vi "PH_PILS.set Doors HV room.vi"(0 "i ref in":refnum<vi>, 2 "Service Name":string="N/A", 5 "error in":errorcluster) -> (14 "i ref out":refnum<vi>, 19 "error out":errorcluster)   [LabVIEW 2014, in "PH_PILS.lvlib"]
doc: "This VI sets the GUI elements related to the doors of the HV room."
uses:
  PH_PILS.lvlib
  PH_PILS.Operation Mode.ctl
  PH_PILS.Submode.ctl
  PH_Basics/PH_Common/PH_Common.lvlib
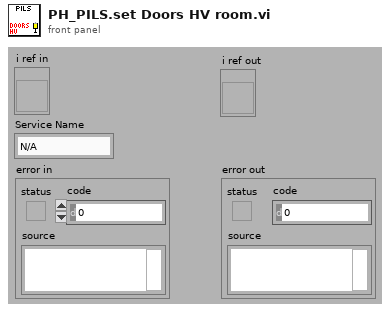
[diagram p1: front panel]
types:
  T1 = typedef "PH_PILS.lvlib/PH_PILS.Submode.ctl" = enum16{"unknown", "HV-Normal", "HV-Test"}
  T2 = typedef "PH_PILS.lvlib/PH_PILS.Operation Mode.ctl" = enum16{"unknown", "Service", "Labor", "Search", "Shot"}
  T3 = typedef "PH_PILS.lvlib/PH_PILS.i attribute.ctl" = cluster{"Boolean":cluster{"GUI Ref":refnum<vi>, "Status":i32}[], "GUI Refs Exp. Shutters":cluster{"1":refnum<vi>, "2":refnum<vi>, "3":refnum<vi>, "4":refnum<vi>}, "Tristate2Run GUI Refs":refnum<vi>[], "EO-Likes":cluster{"GUI Ref":refnum<vi>, "Status":i32}[], "Operation Mode":cluster{"Operation Mode":T2, "GUI":cluster{"Ref State":refnum<vi>, "Ref":refnum<vi>}, "Servicemode":cluster{"Tagname":string, "Status":i32}, "Labormode":cluster{"Tagname":string, "Status":i32}, "Searchmode":cluster{"Tagname":string, "Status":i32}, "Shotmode":cluster{"Tagname":string, "Status":i32}}, "Submode":cluster{"Submode":T1, "GUI":cluster{"Ref State":refnum<vi>, "Ref":refnum<vi>}, "Submode":cluster{"Tagname":string, "Status":i32}}, "Experiment":cluster{"Experiment":enum16{"unknown", "intern", "4 (Z6)", "3", "2", "1"}, "GUI":cluster{"Ref State":refnum<vi>, "Ref":refnum<vi>}, "intern":cluster{"Tagname":string, "Status":i32}, "Exp 4":cluster{"Tagname":string, "Status":i32}, "Exp 3":cluster{"Tagname":string, "Status":i32}, "Exp 2":cluster{"Tagname":string, "Status":i32}, "Exp 1":cluster{"Tagname":string, "Status":i32}}, "TristateNormal":cluster{"GUI Ref":refnum<vi>, "Status":i32}[], "Door Tags":cluster{"GUI Ref":refnum<vi>, "Status":i32}[], "GUIlessTags":cluster{"Name":string, "Status":i32}[], "Beamline GUI Refs":refnum<vi>[], "Special Boolean":cluster{"GUI Ref":refnum<vi>, "Status":i32}[], "Laserpower":cluster{"GUI Ref":refnum<vi>, "Status":i32}[], "Shutter":cluster{"GUI Ref":refnum<vi>, "Status":i32}[], "Tristate EO Like":cluster{"GUI Ref":refnum<vi>, "Status":i32}[], "PP":cluster{"GUI Ref":refnum<vi>, "Status":i32, "Head Ref":refnum<vi>, "Slider Ref":refnum<vi>}[], "Switch Knobs":cluster{"GUI Ref":refnum<vi>, "Status":i32}[], "Latch Knob GUI Refs":refnum<vi>[], "FailureCounter":i32, "Enabled Status":cluster{"Laser":i32, "PreAmp":i32, "MainAmp":i32}, "Mercury":refnum<vi>, "Instance Rods":string, "Logfile":path, "Beckhoff-Instance Internal":string, "Beckhoff-Instance External":string, "Enabling Rights":cluster{"Name":string, "Password":string, "PA?":bool, "MA?":bool, "Exp?":bool}[]}
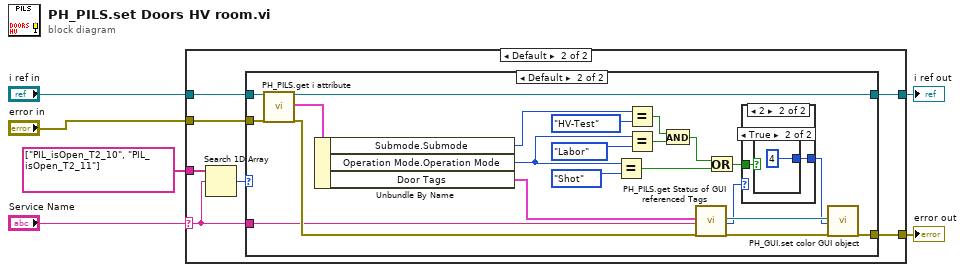
[diagram p0: block diagram]
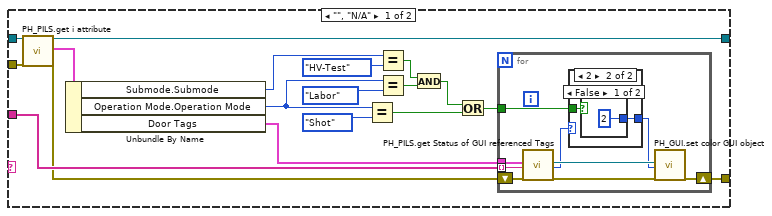
[diagram p2: hidden frame]
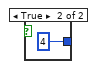
[diagram p4: hidden frame]
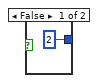
[diagram p7: hidden frame]
diagram:
  n1 = case shown="Default" "Service Name" {
    selector: "Service Name" -> [_ w40]
    tunnel: "error in" -> [w24 w45]
    tunnel: [w23 w44] -> w5
    tunnel: "i ref in" -> [w22 w43]
    tunnel: [w20 w42] -> w3
    tunnel: string[] ["PIL_isOpen_T2_10", "PIL_isOpen_T2_11"] -> [w19 w41]
    frame "", "N/A" {
      n2 = call "PH_PILS.get i attribute.vi"("i ref in"=w22, "error in (no error)"=w24) -> ("i ref out"=w23:refnum<vi>, "i attribute"=w21:T3, "error out"=w16:errorcluster)  [unwired: 15 in]
      n3 = Unbundle By Name(w21) -> ("Submode.Submode"=w13:T1, "Operation Mode.Operation Mode"=w14:T2, "Door Tags"=w17:cluster{"GUI Ref":refnum<vi>, "Status":i32}[])
      n4 = Equal?(x=w14, y=PH_PILS.Operation_Mode."Shot" ("Operation Mode.Operation Mode")) -> (x = y?=w8:bool)
      n5 = Equal?(x=w13, y=PH_PILS.Submode."HV-Test" ("Submode.Submode")) -> (x = y?=w11:bool)
      n6 = Equal?(x=w14, y=PH_PILS.Operation_Mode."Labor" ("Operation Mode.Operation Mode")) -> (x = y?=w10:bool)
      n7 = And(x=w11, y=w10) -> (x .and. y?=w9:bool)
      n8 = Or(x=w9, y=w8) -> (x .or. y?=w7:bool)
      n9 = for {
        tunnel: w17 -> [w33]
        tunnel: w19 -> [w30] mode=indexing
        shift-right: [w29] -> w20
        shift-left: w16 -> [w32]
        tunnel: w7 -> [w25]
        n10 = call "PH_PILS.get Status of GUI referenced Tags.vi"("Tags"=w33, "Tagname"=w30, "error in"=w32) -> ("GUI Ref"=w28:refnum<vi>, "Status"=w27:i32, "error out"=w31:errorcluster)  [unwired: 13 in, 1 out]
        n11 = case shown="2" w27 {
          selector: w27 -> [w34 _]
          tunnel: [w34 w36] -> w26
          tunnel: w25 -> [_ w35]
          frame 0, Default {
          }
          frame 2 {
            n12 = case shown="False" w35 {
              tunnel: [2 4] -> w36
              frame False {
              }
              frame True {
              }
            }
          }
        }
        n13 = call "PH_GUI.set color GUI object.vi"("GUI object Ref"=w28, "State"=w26, "error in (no error)"=w31) -> ("error out"=w29:errorcluster)  [unwired: 16 in]
      }
    }
    frame Default {
      n14 = Search 1D Array(1D array=w41, element=w40) -> (index of element=w39:i32)  [unwired: 1 in]
      n15 = case shown="Default" w39 {
        tunnel: w45 -> [w46 w69]
        tunnel: [w47 w68] -> w44
        tunnel: w43 -> [w47 w67]
        tunnel: [w46 w65] -> w42
        tunnel: w40 -> [_ w52]
        frame -1 {
        }
        frame Default {
          n16 = call "PH_PILS.get i attribute.vi"("i ref in"=w67, "error in (no error)"=w69) -> ("i ref out"=w68:refnum<vi>, "i attribute"=w66:T3, "error out"=w62:errorcluster)  [unwired: 15 in]
          n17 = Unbundle By Name(w66) -> ("Submode.Submode"=w59:T1, "Operation Mode.Operation Mode"=w60:T2, "Door Tags"=w63:cluster{"GUI Ref":refnum<vi>, "Status":i32}[])
          n18 = Equal?(x=w60, y=PH_PILS.Operation_Mode."Shot" ("Operation Mode.Operation Mode")) -> (x = y?=w54:bool)
          n19 = Equal?(x=w59, y=PH_PILS.Submode."HV-Test" ("Submode.Submode")) -> (x = y?=w57:bool)
          n20 = Equal?(x=w60, y=PH_PILS.Operation_Mode."Labor" ("Operation Mode.Operation Mode")) -> (x = y?=w56:bool)
          n21 = And(x=w57, y=w56) -> (x .and. y?=w55:bool)
          n22 = call "PH_PILS.get Status of GUI referenced Tags.vi"("Tags"=w63, "Tagname"=w52, "error in"=w62) -> ("GUI Ref"=w50:refnum<vi>, "Status"=w49:i32, "error out"=w51:errorcluster)  [unwired: 13 in, 1 out]
          n23 = Or(x=w55, y=w54) -> (x .or. y?=w53:bool)
          n24 = case shown="2" w49 {
            selector: w49 -> [w70 _]
            tunnel: [w70 w72] -> w48
            tunnel: w53 -> [_ w71]
            frame 0, Default {
            }
            frame 2 {
              n25 = case shown="True" w71 {
                tunnel: [2 4] -> w72
                frame False {
                }
                frame True {
                }
              }
            }
          }
          n26 = call "PH_GUI.set color GUI object.vi"("GUI object Ref"=w50, "State"=w48, "error in (no error)"=w51) -> ("error out"=w65:errorcluster)  [unwired: 16 in]
        }
      }
    }
  }
  "error out" <- w3
  "i ref out" <- w5
